vi "Bead Recorder.vi"() -> ()   [LabVIEW 2021]
uses:
  Hardware Configuration/Hardware Configuration Controls/Device Type.ctl
  Hardware Configuration/Hardware Configuration Controls/Device Function.ctl
  Device Library/Stages/Stages Controls/Stage Actions.ctl
  4Pi Capture Manager - DM/4Pi Capture Manager Controls/4Pi Capture Notifier Type.ctl
  4Pi Capture Manager - DM/4Pi Capture Manager Controls/4Pi Capture Actions.ctl
  4Pi Capture Manager - DM/4Pi Capture Manager Controls/4Pi Capture Switch Line Scan Modes.ctl
  4Pi Capture Manager - DM/4Pi Capture Manager Controls/DM scan mode.ctl
  4Pi Dual DM Control/4Pi Dual DM - Controls/4Pi Dual DM - Mirror Modes.ctl
panel:
  in  "wait time (s)":dbl
  in  "Quit":bool
  in  "Record":bool
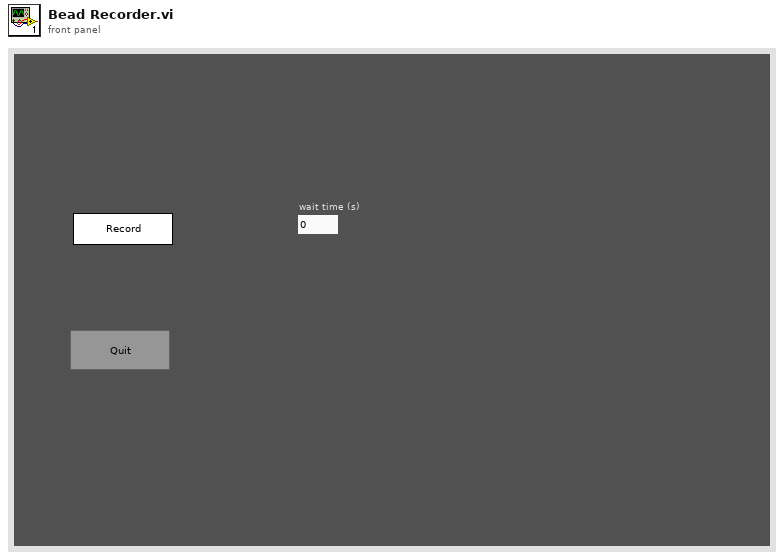
[diagram p1: front panel]
types:
  T1 = typedef "4Pi Capture Notifier Type.ctl" = cluster{"Actions":T2, "Running?":bool, "Preview Exposure (s)":dbl, "Capture Exposure (s)":dbl, "Cycles":u16, "Frames":u32, "No. of Z Steps":u16, "Z Step Size (µm)":dbl, "Base Path":path, "Init Z Position (µm)":dbl, "Lasers Lines":string[], "Save Path":path, "Line Scan?":bool, "Line Scan Mode":T3, "No. Amp steps":u16, "Amp step size":dbl, "No. Mirror Mode":u16, "DM scan mode":T4, "Metadata File Ref":refnum<file>[], "Init Mirror Modes":T5, "Sampling Time (s)":dbl}
  T2 = typedef "4Pi Capture Actions.ctl" = enum16{"Idle", "Live Preview", "Capture", "Laser On", "Laser Off", "Open Shutters", "Close Shutters", "Set Exposure Time", "Start Acquisition", "Update SubFolder", "Setup", "Camera Soft Trigger", "Camera", "Swtich1", "Switch", "Step", "Cycle", "Write DM", "External Cycle Sync", "Write Metadata", "Abort", "Quit"}
  T3 = typedef "4Pi Capture Switch Line Scan Modes.ctl" = enum32{"Automatic", "Use Presets", "Manual"}
  T4 = typedef "DM scan mode.ctl" = u16
  T5 = typedef "4Pi Dual DM - Mirror Modes.ctl" = cluster{"Mode":string, "Amplitude":dbl}[]
  T6 = typedef "Stage Actions.ctl" = enum16{"Get Position", "SERVO OFF", "SERVO ON", "SERVO ON/OFF", "MVR", "MOVE", "HALT", "ONTARGET", "ERROR", "REFERENCE", "INIT", "VELOCITY", "STATUS", "EXIT", "HOME", "ZEROPOS", "NANOPOS", "ANALOG", "QUIT"}
  T7 = typedef "Device Function.ctl" = enum16{"Primary", "Secondary", "Overview", "Wide Field Drift Correction", "642 nm Excitation", "560 nm Excitation", "940 nm Excitation", "546 nm Excitation", "488 nm Excitation", "405 nm Excitation", "Objective Drift Correction", "4Pi Focus Lock", "4Pi Objective Lock", "Objective XY", "Objective Z", "Sample XY", "Sample Coarse Z", "Sample Z", "4Pi Lower", "4Pi Upper", "Em Small", "Em Large", "Ex Small", "Ex Large", "Mojo", "Adj Cavity", "Line Scanning", "Alert"}
  T8 = typedef "Device Type.ctl" = enum16{"AOTF", "Camera", "Deformable Mirror", "Laser", "Flip Mirror", "Shutter", "Stage", "Waveform", "FPGA", "Email"}
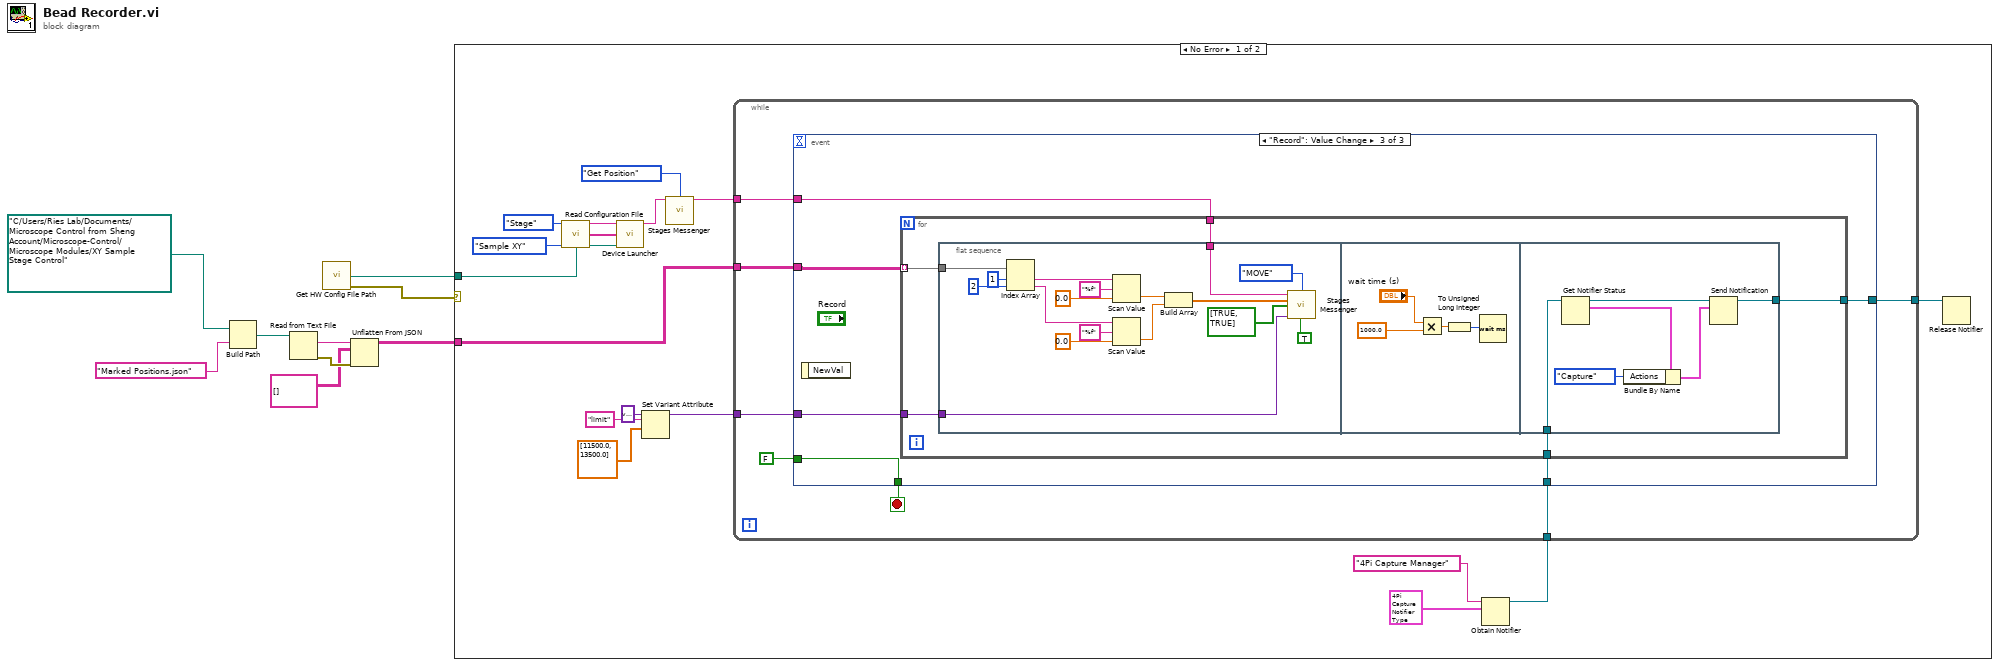
[diagram p0: block diagram]
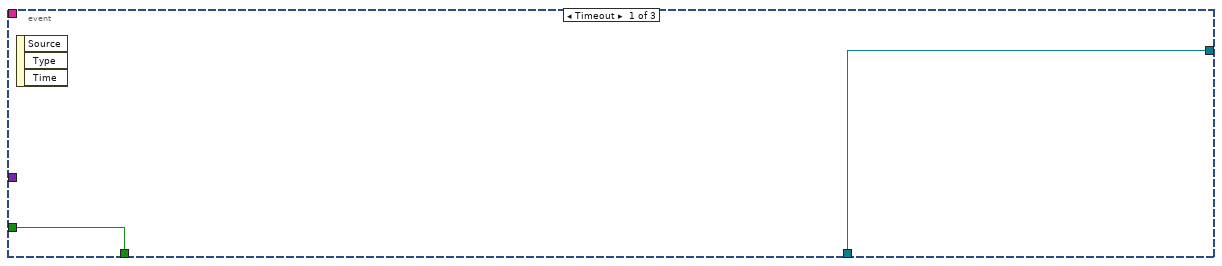
[diagram p2: hidden frame]
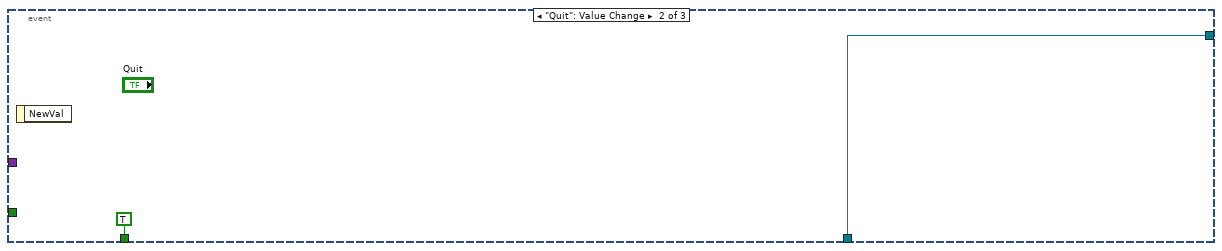
[diagram p3: hidden frame]
diagram:
  n1 = Build Path(base path=path "C:/Users/Ries Lab/Documents/Microscope Control from Sheng Account/Microscope-Control/Microscope Modules/XY Sample Stage Control" ("path"), name or relative path="Marked Positions.json") -> (appended path=w3:path)
  n2 = Read from Text File(file (use dialog)=w3) -> (text=w6:string, error out=w5:errorcluster)  [unwired: 3 in, 2 out]
  n3 = call "Get HW Config File Path.vi"() -> ("File Path"=w8:path, "Error"=w9:errorcluster)  [unwired: 14 in]
  n4 = Unflatten From JSON(JSON string=w6, type and defaults=string[][] [] ("Item Names"), error in (no error)=w5) -> (value=w1:string[][])  [unwired: 4 in, 1 out]
  n5 = case shown="No Error" w9 {
    tunnel: w8 -> [w22 _]
    tunnel: w1 -> [w18 _]
    frame No Error {
      n6 = call "Read Configuration File.vi"("Device Type"=Device_Type."Stage", "Device Function"=Device_Function."Sample XY", "Config File Path"=w22) -> ("Unique Notifier Name"=w27:string, "Device Ports/IDs/Channels"=w25:string[], "Device Engine Path"=w26:path)  [unwired: 9 in, 1 out]
      n7 = call "Device Launcher.vi"("Notifier Name"=w27, "Device Ports/IDs/Channels"=w25, "Device Engine Path"=w26) -> ("Notifier Name"=w21:string)  [unwired: 11 in, 1 out]
      n8 = Set Variant Attribute(Variant=variant ("variant"), name="limit", value=dbl[] [11500.0, 13500.0] ("Array")) -> (Variant out=w10:variant)  [unwired: 1 in, 2 out]
      n9 = call "Stages Messenger.vi"("Stage Notifier Name"=w21, "Actions"=Stage_Actions."Get Position") -> ("Stage Notifier Name (Dup)"=w19:string)  [unwired: 9 in, 4 out]
      n10 = Obtain Notifier(name (unnamed)="4Pi Capture Manager", notification data type=T1 {"Actions"=enum."Live Preview", "Running?"=FALSE, "Preview Exposure (s)"=0.1, "Capture Exposure (s)"=0.1, "Cycles"=1, "Frames"=0, "No. of Z Steps"=0, "Z Step Size (µm)"=0.0, "Base Path"=path "", "Init Z Position (µm)"=0.0, "Lasers Lines"=[], "Save Path"=path "", "Line Scan?"=FALSE, "Line Scan Mode"=enum."Automatic", "No. Amp steps"=0, "Amp step size"=0.0, "No. Mirror Mode"=0, "DM scan mode"=0, "Metadata File Ref"=[], "Init Mirror Modes"=[], "Sampling Time (s)"=0.0} ("4Pi Capture Notifier Type")) -> (notifier out=w14:refnum<notifier>)  [unwired: 2 in, 2 out]
      n11 = while {
        tunnel: w18 -> [w33]
        tunnel: [w32] -> w17
        tunnel: w19 -> [w34]
        tunnel: w14 -> [w29]
        tunnel: w10 -> [w28]
        stop <- w31 stop-if-true
        n12 = event shown="[2] \"Record\": Value Change" {
          selector: _ -> [_ _ _]
          dyn-events: _ -> [_ _ _]
          timeout: _ -> [_ _ _]
          tunnel: w34 -> [_ _ w41]
          tunnel: w33 -> [_ _ w44]
          tunnel: [w35 w37 w43] -> w32
          tunnel: FALSE ("NewVal") -> [w36 _ w42]
          tunnel: [w36 TRUE ("NewVal") w42] -> w31
          tunnel: w29 -> [w35 w37 w40]
          tunnel: w28 -> [_ _ w39]
          event Timeout {
            n13 = event-data() -> ()  [unwired: 1 in, 3 out]
          }
          event "Quit": Value Change {
            n14 = event-data() -> ()  [unwired: 1 in, 1 out]
          }
          event "Record": Value Change {
            n15 = event-data() -> ()  [unwired: 1 in, 1 out]
            n16 = for {
              tunnel: w44 -> [w49] mode=indexing
              tunnel: w41 -> [w48]
              tunnel: [w47] -> w43
              tunnel: w40 -> [w46]
              tunnel: w39 -> [w45]
              n17 = flat-sequence {
                tunnel: w49 -> [w52]
                tunnel: w48 -> [w51]
                tunnel: w45 -> [w50]
                tunnel: [w72] -> w47
                tunnel: w46 -> [w71]
                frame #0 {
                  n18 = Index Array(array=w52, index #1=1 ("index"), index #2=2 ("index")) -> (element #1=w57:string, element #2=w53:string)
                  n19 = Scan Value(string=w57, format string="%f", default (0 dbl)=0.0) -> (value=w56:dbl)  [unwired: 1 out]
                  n20 = Scan Value(string=w53, format string="%f", default (0 dbl)=0.0) -> (value=w55:dbl)  [unwired: 1 out]
                  n21 = Build Array(w56, w55) -> (w54:dbl[])
                  n22 = call "Stages Messenger.vi"("Stage Notifier Name"=w51, "Actions"=Stage_Actions."MOVE", "Setpoint"=w54, "Axis"=bool[] [TRUE, TRUE], "Misc"=w50, "Exit While Busy?"=TRUE ("Wait for On Target? (F)")) -> ()  [unwired: 5 in, 5 out]
                }
                frame #1 {
                  n23 = Multiply(x="wait time (s)", y=1000.0) -> (x*y=w68:dbl)
                  n24 = To Unsigned Long Integer(number=w68) -> (unsigned 32bit integer=w67:u32)
                  n25 = Wait (ms)(milliseconds to wait=w67) -> ()  [unwired: 1 out]
                }
                frame #2 {
                  n26 = Get Notifier Status(notifier=w71) -> (notifier out=w76:refnum<notifier>, current notification=w75:T1)  [unwired: 1 in, 3 out]
                  n27 = Bundle By Name(cluster=w75, "Actions"=4Pi_Capture_Actions."Capture") -> (w73:T1)
                  n28 = Send Notification(notification=w73, notifier=w76) -> (notifier out=w72:refnum<notifier>)  [unwired: 1 in, 1 out]
                }
              }
            }
          }
        }
      }
      n29 = Release Notifier(notifier=w17) -> ()  [unwired: 2 in, 3 out]
    }
    frame Error {
    }
  }
